vi "Load Init Configuration (SubVI).vi"() -> (0 "error out":errorcluster, 3 "datafolder":path)   [LabVIEW 2020, in "FileIO.lvlib"]
uses:
  FileIO.lvlib
  <vilib>/Utility/config.llb/Read Key (Path).vi
  <vilib>/Utility/config.llb/NI_LVConfig.lvlib
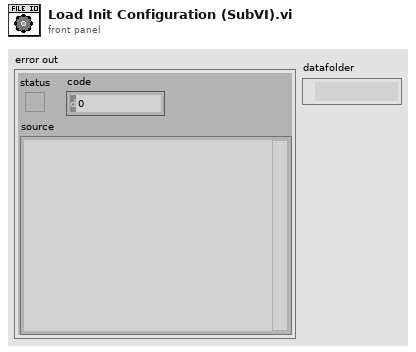
[diagram p1: front panel]
types:
  T1 = typedef "NI_LVConfig.lvlib/Config Data RefNum.ctl" = refnum<k1>
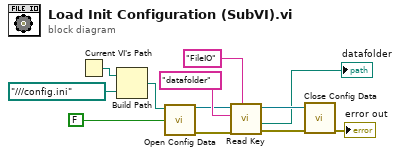
[diagram p0: block diagram]
diagram:
  n1 = Current VI's Path() -> (path=w3:path)
  n2 = Build Path(base path=w3, name or relative path=path "../../../config.ini" ("configuration file path")) -> (appended path=w1:path)
  n3 = call <vilib>:"Open Config Data.vi"("create file if necessary (T)"=FALSE, "configuration file path"=w1) -> ("error out"=w9:errorcluster, "refnum"=w11:T1)  [unwired: 7 in, 1 out]
  n4 = call-poly <vilib>:"Read Key.vi"("section"="FileIO", "error in (no error)"=w9, "key"="datafolder", "refnum"=w11) -> ("error out"=w8:errorcluster, "value"=→"datafolder":path, "refnum out"=w7:T1)  [unwired: 4 in, 1 out]
  n5 = call <vilib>:"Close Config Data.vi"("error in (no error)"=w8, "refnum"=w7) -> ("error out"=→"error out":errorcluster)  [unwired: 8 in, 1 out]
